vi "SAOccupiedBandwidthTraceFetch.vi"(8 "error in (no error)":errorcluster {"code" format="%.0x"}, 9 "RetValBufferSize":i32=2048 caption="RetValBufferSize (2048)", 10 "RepCapIdentifier":string="OCB_Results" caption="RepCapIdentifier (OCB_Results)", 11 "instrument handle":refnum<k15>) -> (0 "error out":errorcluster {"code" format="%.0x"}, 1 "RetValActualSize":i32, 2 "RetVal":dbl[](array[numeric]) format="%.2p", 3 "instrument handle out":refnum<k15>)   [LabVIEW 2009, in "Keysight XSAn.lvlib"]
doc: "Puts selected data from the most recent measurement into the output buffer.\n\nSupported Models: M9290A, N8973B, N8974B, N8975B, N8976B, N9000A, N9000B, N9010A, N9010B, N9020A, N9020B, N9030A, N9030B, N9038A, N9040B, N9041B, SPN9003A, SPN9026A"
uses:
  <instrlib>/Keysight XSAn/Keysight XSAn.lvlib
  AgXSAn.dll
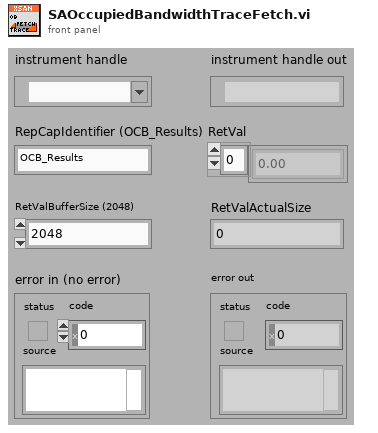
[diagram p1: front panel]
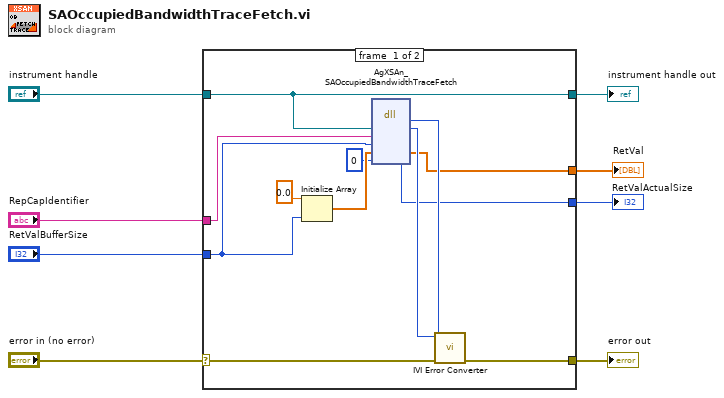
[diagram p0: block diagram]
diagram:
  n1 = case shown="No Error" "error in (no error)" {
    selector: "error in (no error)" -> [w18 w22]
    tunnel: [w17 w22] -> w8
    tunnel: "instrument handle" -> [w10 w21]
    tunnel: "RepCapIdentifier" -> [w16 _]
    tunnel: "RetValBufferSize" -> [w9 _]
    tunnel: [w13 _] -> w3
    tunnel: [w11 _] -> w2
    tunnel: [w10 w21] -> w1
    frame #0 {
      n2 = Initialize Array(0.0 ("element"), w9) -> (w15:dbl[])
      n3 = dll-call lib="AgXSAn**.dll" fn="AgXSAn_SAOccupiedBandwidthTraceFetch"("Vi"=w10, "RepCapIdentifier"=w16, "RetValBufferSize"=w9, "RetVal"=w15, "RetValActualSize"=0) -> (w19:i32, "Vi"=w20:u32, "RetVal"=w13:dbl[], "RetValActualSize"=w11:i32)  [unwired: 5 in, 2 out]
      n4 = call <instrlib>:"IVI Error Converter.vi"("error in (no error)"=w18, "IVI error code (0)"=w19, "instrument handle"=w20) -> ("error out"=w17:errorcluster)  [unwired: 7 in, 1 out]
    }
    frame #1 {
    }
  }
  "error out" <- w8
  "instrument handle out" <- w1
  "RetVal" <- w3
  "RetValActualSize" <- w2
